vi "sub_NMEAstr-2-latlon.vi"(10 "문자열":string, 11 "문자열 2":string) -> (3 "클러스터":cluster{"lat":dbl, "lon":dbl})   [LabVIEW 2019]
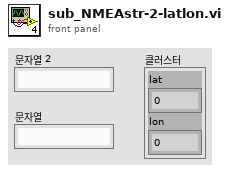
[diagram p1: front panel]
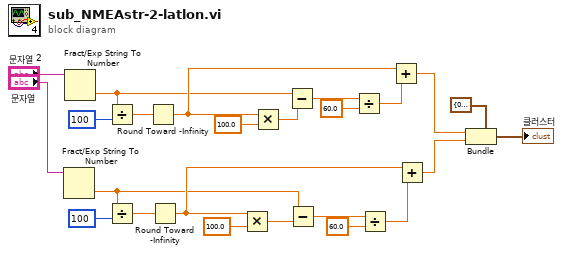
[diagram p0: block diagram]
diagram:
  n1 = Fract/Exp String To Number(string="문자열") -> (number=w10:dbl)  [unwired: 3 in, 1 out]
  n2 = Fract/Exp String To Number(string="문자열 2") -> (number=w9:dbl)  [unwired: 3 in, 1 out]
  n3 = Divide(x=w9, y=100) -> (x/y=w5:dbl)
  n4 = Divide(x=w10, y=100) -> (x/y=w8:dbl)
  n5 = Round Toward -Infinity(1:w5) -> (0:w17:dbl)
  n6 = Round Toward -Infinity(1:w8) -> (0:w19:dbl)
  n7 = Multiply(x=w19, y=100.0) -> (x*y=w7:dbl)
  n8 = Multiply(x=w17, y=100.0) -> (x*y=w6:dbl)
  n9 = Subtract(x=w9, y=w6) -> (x-y=w12:dbl)
  n10 = Subtract(x=w10, y=w7) -> (x-y=w15:dbl)
  n11 = Divide(x=w12, y=60.0) -> (x/y=w16:dbl)
  n12 = Divide(x=w15, y=60.0) -> (x/y=w18:dbl)
  n13 = Add(x=w17, y=w16) -> (x+y=w20:dbl)
  n14 = Add(x=w19, y=w18) -> (x+y=w21:dbl)
  n15 = Bundle(cluster=cluster{"lat":dbl, "lon":dbl} {"lat"=0.0, "lon"=0.0} ("클러스터"), "lat"=w20, "lon"=w21) -> (→"클러스터":cluster{"lat":dbl, "lon":dbl})
